vi "Delete All Attributes.vi"(7 "Tree ID":string, 8 "Error In":errorcluster, 11 "Tree Manager":T1) -> (0 "Error Out":errorcluster, 3 "Tree Manager":T1)   [LabVIEW 2020, in "NI_VIAnCFGDataStructure.lvlib" / "Tree.lvclass"]
doc: "Delete all variant attributes from the Tree."
uses:
  <vilib>/addons/analyzer/VIAnCFGDataStructure/Tree Manager/Tree.lvclass
  <vilib>/addons/analyzer/VIAnCFGDataStructure/Tree Manager/Typedefs/Session Handle.ctl
  <vilib>/addons/analyzer/VIAnCFGDataStructure/Tree Manager/Tree.lvclass/Tree.ctl
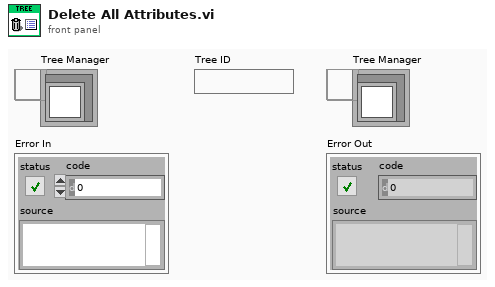
[diagram p1: front panel]
types:
  T1 = typedef "NI_VIAnCFGDataStructure.lvlib/Tree.lvclass/Session Handle.ctl" = refnum<data-value>
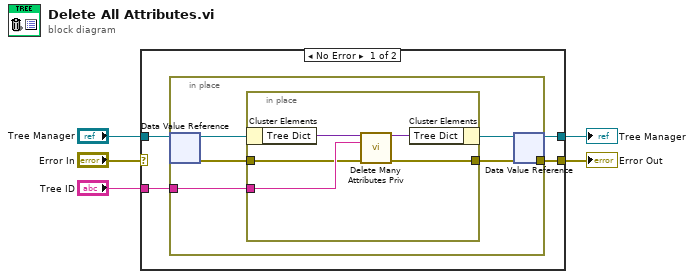
[diagram p0: block diagram]
diagram:
  n1 = case shown="No Error" "Error In" {
    selector: "Error In" -> [_ w20]
    tunnel: "Tree Manager" -> [w9 w21]
    tunnel: [w8 w21] -> w4
    tunnel: [w7 w20] -> w2
    tunnel: "Tree ID" -> [w6 _]
    frame No Error {
      n2 = in-place {
        in-place-border: [w13] -> w7
        in-place-border: w6 -> [w11]
        n3 = in-place-dvr #1(w9) -> (w14:refnum<class "Tree.lvclass">, w10:errorcluster)
        n4 = in-place {
          in-place-border: [w17] -> w13
          in-place-border: w11 -> [w18]
          in-place-border: w10 -> [w15]
          n5 = in-place-cluster #2(w14) -> ("Tree Dict"=w19:variant)
          n6 = call <vilib>:"Delete Many Attributes Priv.vi"("Tree Dictionary In"=w19, "Unique ID"=w18, "error in"=w15) -> ("Tree Dictionary Out"=w16:variant, "error out"=w17:errorcluster)  [unwired: 11 in]
          n7 = in-place-cluster #2("Tree Dict"=w16) -> (w12:refnum<class "Tree.lvclass">)
        }
        n8 = in-place-dvr #1(w12) -> (w8:T1)  [unwired: 1 out]
      }
    }
    frame Error {
    }
  }
  "Tree Manager" <- w4
  "Error Out" <- w2
